vi "G4SubTemplate_Singleton_6x8x6_WriteAttribute.vi"(5 "error in (no error)":errorcluster) -> (19 "error out":errorcluster)   [LabVIEW 2014]
uses:
  <resource>/Framework/Providers/Open_GDS/ClassProviders/Provider_EndevoGOOP400/Templates/G4SubTemplate_Singleton_6x8x6/G4SubTemplate_Singleton_6x8x6.lvclass
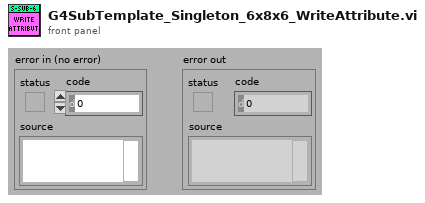
[diagram p1: front panel]
types:
  T1 = typedef "G4SubTemplate_Singleton_6x8x6.lvclass/ObjectAttributes.ctl" = cluster{"Attribute1":dbl}
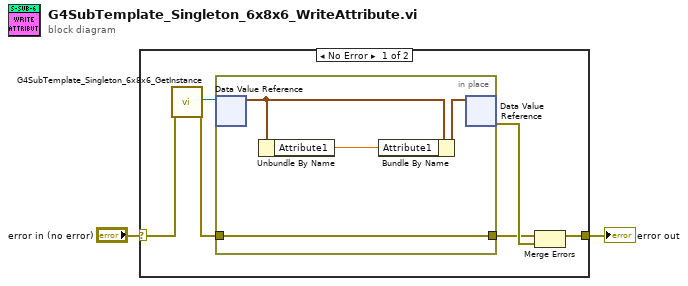
[diagram p0: block diagram]
diagram:
  n1 = case shown="No Error" "error in (no error)" {
    selector: "error in (no error)" -> [w6 w13]
    tunnel: [w7 w13] -> w1
    frame No Error {
      n2 = call <resource>:"G4SubTemplate_Singleton_6x8x6_GetInstance.vi"("error in (no error)"=w6) -> ("DVRRefOut"=w5:refnum<data-value>, "error out"=w4:errorcluster)  [unwired: 14 in, 3 out]
      n3 = in-place {
        in-place-border: w4 -> [w11]
        in-place-border: [w11] -> w3
        n4 = in-place-dvr #1(w5) -> (w10:T1)  [unwired: 1 out]
        n5 = Unbundle By Name(w10) -> ("Attribute1"=w9:dbl)
        n6 = Bundle By Name(cluster=w10, "Attribute1"=w9) -> (w12:T1)
        n7 = in-place-dvr #1(w12) -> (w8:errorcluster)  [unwired: 1 out]
      }
      n8 = Merge Errors(w3, w8) -> (w7:errorcluster)
    }
    frame Error {
    }
  }
  "error out" <- w1
